vi "runscenario process Conditions.vi"(8 "error in (no error)":errorcluster, 10 "Conditions (none)":T3[](array[typedef]), 11 "Connection Refnum":T1) -> (0 "error out":errorcluster, 1 "Test Run Filter":string, 2 "Conditions":T2, 3 "dup Connection Refnum":T1)   [LabVIEW 2011]
uses:
  server/database/Scenarios/Conditions/Condition Record.ctl
  server/database/Scenarios/Conditions/Condition Operators.ctl
  Addons/internet/utils/keyedarr.llb/Keyed Array.ctl
  SI.LIB/ODBC/SQL Controls/Connection Refnum.ctl
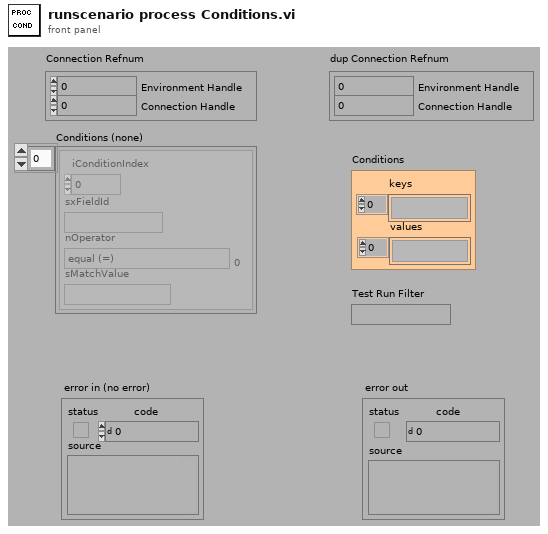
[diagram p1: front panel]
types:
  T1 = typedef "Connection Refnum.ctl" = cluster{"Environment Handle":i32, "Connection Handle":i32}
  T2 = typedef "Keyed Array.ctl" = cluster{"keys":string[], "values":string[]}
  T3 = typedef "Condition Record.ctl" = cluster{"iConditionIndex":i32, "sxFieldId":string, "nOperator":T4, "sMatchValue":string}
  T4 = typedef "Condition Operators.ctl" = enum16{"equal (=)", "not equal (\\u2260)", "less than (<)", "less than or equal (\\u2264)", "greater than (>)", "greater than or equal (\\u2265)", "contains", "does not contain"}
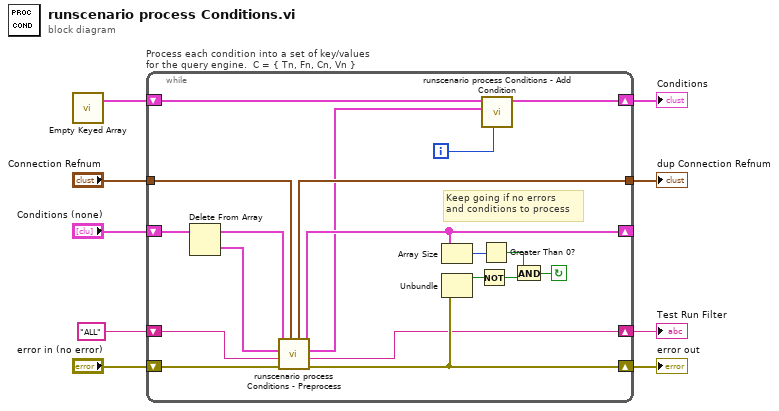
[diagram p0: block diagram]
diagram:
  n1 = call "Empty Keyed Array.vi"() -> ("empty keyed array"=w9:T2)  [unwired: 3 out]
  n2 = while "Process each condition into a set of key/values for the query engine.  C = { Tn, Fn, Cn, Vn }" {
    shift-right: [w21] -> w8
    shift-left: w9 -> [w22]
    shift-right: [w11] -> w7
    shift-left: "ALL" ("key") -> [w12]
    shift-right: [w17] -> w3
    shift-left: "error in (no error)" -> [w20]
    tunnel: "Connection Refnum" -> [w16]
    shift-right: [w18] -> _
    shift-left: "Conditions (none)" -> [w28]
    tunnel: [w15] -> w1
    i -> [w10]
    stop <- w25 continue-if-true
    # "Keep going if no errors\nand conditions to process"
    n3 = Delete From Array(array=w28) -> (deleted portion=w14:T3, array with subset deleted=w19:T3[])  [unwired: 2 in]
    n4 = call "runscenario process Conditions - Preprocess.vi"("Connection Refnum"=w16, "error in (no error)"=w20, "Run Filter (\"\")"=w12, "Condition"=w14, "Condition Stack (empty)"=w19) -> ("error out"=w17:errorcluster, "new Run Filter"=w11:string, "Condition out"=w13:T3, "Condition Stack"=w18:T3[], "dup Connection Refnum"=w15:T1)  [unwired: 2 out]
    n5 = Array Size(array=w18) -> (size(s)=w27:i32)
    n6 = Unbundle(w17) -> ("status"=w23:bool)  [unwired: 2 out]
    n7 = Not(x=w23) -> (.not. x?=w24:bool)
    n8 = Greater Than 0?(x=w27) -> (x > 0?=w26:bool)
    n9 = call "runscenario process Conditions - Add Condition.vi"("Condition Count (0)"=w10, "Condition"=w13, "Conditions (empty)"=w22) -> ("Conditions"=w21:T2)  [unwired: 1 in, 7 out]
    n10 = And(x=w26, y=w24) -> (x .and. y?=w25:bool)
  }
  "Conditions" <- w8
  "Test Run Filter" <- w7
  "error out" <- w3
  "dup Connection Refnum" <- w1
